vi "Convert Unit Circle to Radians.vi"(11 "Unit Circle":dbl) -> (3 "Radians":dbl)   [LabVIEW 2023, in "TShirtWork-SwerveDrive_ACT_ts.lvlib"]
uses:
  TShirtWork-SwerveDrive_ACT_ts.lvlib
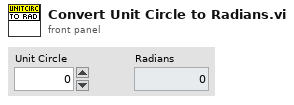
[diagram p1: front panel]
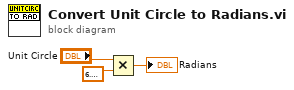
[diagram p0: block diagram]
diagram:
  n1 = Multiply(x="Unit Circle", y=6.283185307179586) -> (x*y=→"Radians":dbl)
